vi "expodrive.vi"(10 "Input 2":dbl, 11 "Input":dbl) -> (2 "Output 2":dbl, 3 "Output":dbl)   [LabVIEW 2010, in "LASA Beta.lvrbt"]
uses:
  LASA Beta.lvrbt
  <vilib>/NXT/Dual Mode Library/prims/inRangeAndCoerce/inRangeAndCoerce_int.vi
  <vilib>/NXT/Dual Mode Library/prims/inRangeAndCoerce/inRangeAndCoerce_float.vi
panel:
  in  "Last Sign 2":i32
  in  "Last Sign":i32
  in  "Time 2":i32
  in  "Time 1":i32
  in  "Last Time 2":u32
  in  "Last Time":u32
  # "Time since last update"
  # "Time (ms)"
  # "Last Direction Moved"
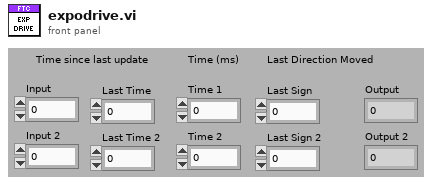
[diagram p1: front panel]
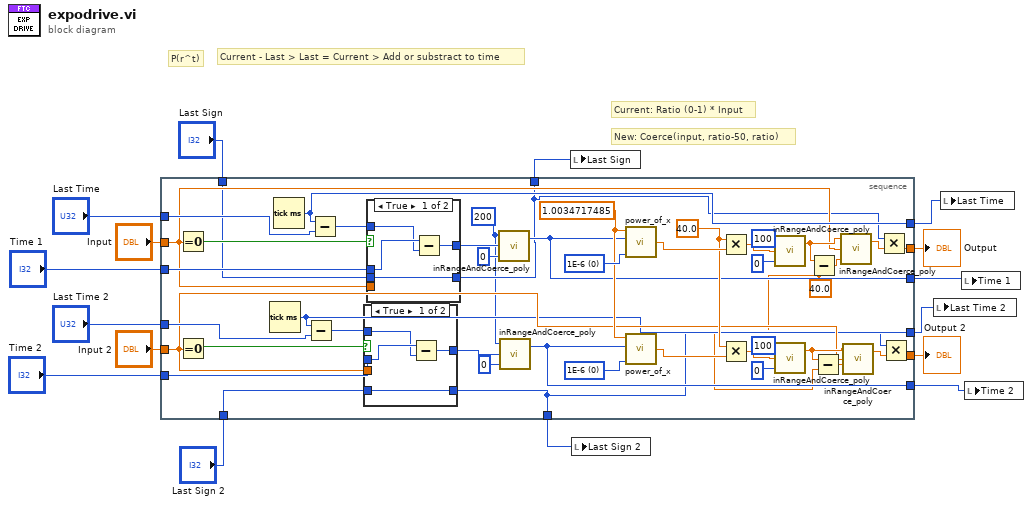
[diagram p0: block diagram]
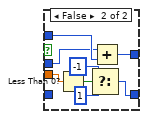
[diagram p2: hidden frame]
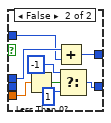
[diagram p3: hidden frame]
diagram:
  # "New: Coerce(input, ratio-50, ratio)"
  # "Current: Ratio (0-1) * Input"
  # "Current - Last > Last = Current > Add or substract to time"
  # "P(r^t)"
  n1 = stacked-sequence {
    tunnel: "Input" -> [w24]
    tunnel: "Input 2" -> [w25]
    tunnel: "Last Time" -> [w47]
    tunnel: [w45] -> w2
    tunnel: "Time 1" -> [w44]
    tunnel: "Last Time 2" -> [w34]
    tunnel: "Time 2" -> [w40]
    tunnel: [w37] -> w4
    tunnel: [w36] -> w3
    tunnel: [w26] -> w10
    tunnel: [w27] -> w9
    tunnel: "Last Sign" -> [w23]
    tunnel: "Last Sign 2" -> [w22]
    tunnel: [w20] -> w6
    tunnel: [w19] -> w5
    tunnel: [w21] -> w1
    frame #0 {
      w17 = 40.0 ("y")
      w18 = 200 ("upper limit")
      w51 = u16 0 items=["1E-6", "1E-5", "1E-4", "1E-3", "1E-2", "1E-1", ""] ("Precision")
      w49 = 40.0
      w56 = u16 0 items=["1E-6", "1E-5", "1E-4", "1E-3", "1E-2", "1E-1", ""] ("Precision")
      w48 = 1.0034717485
      n2 = Equal To 0?(x=w24) -> (x = 0?=w60:bool)
      n3 = Equal To 0?(x=w25) -> (x = 0?=w41:bool)
      n4 = Tick Count (ms)() -> (millisecond timer value=w21:u32)
      n5 = Tick Count (ms)() -> (millisecond timer value=w45:u32)
      n6 = Subtract(x=w21, y=w34) -> (x-y=w35:u32)
      n7 = Subtract(x=w45, y=w47) -> (x-y=w46:u32)
      n8 = case shown="True" w41 {
        tunnel: w35 -> [w63 w72]
        tunnel: w40 -> [w64 w70]
        tunnel: [w62 w71] -> w38
        tunnel: w25 -> [_ w69]
        tunnel: w22 -> [w61 _]
        tunnel: [w61 w65] -> w19
        frame True {
          n9 = Subtract(x=w64, y=w63) -> (x-y=w62:u32)
        }
        frame False {
          n10 = Less Than 0?(x=w69) -> (x < 0?=w68:bool)
          n11 = Select(t=-1, s=w68, f=1) -> (s? t:f=w65:i32)
          n12 = Add(x=w70, y=w72) -> (x+y=w71:u32)
        }
      }
      n13 = case shown="True" w60 {
        tunnel: w46 -> [w75 w83]
        tunnel: w44 -> [w76 w84]
        tunnel: [w74 w82] -> w43
        tunnel: w24 -> [_ w80]
        tunnel: w23 -> [w73 _]
        tunnel: [w73 w79] -> w20
        frame True {
          n14 = Subtract(x=w76, y=w75) -> (x-y=w74:u32)
        }
        frame False {
          n15 = Less Than 0?(x=w80) -> (x < 0?=w81:bool)
          n16 = Add(x=w84, y=w83) -> (x+y=w82:u32)
          n17 = Select(t=-1, s=w81, f=1) -> (s? t:f=w79:i32)
        }
      }
      n18 = call-poly <vilib>:"inRangeAndCoerce_poly.vi"("lower limit"=0, "x"=w43, "upper limit"=w18) -> ("coerced(x)"=w36:i32)  [unwired: 1 out]
      n19 = call-poly <vilib>:"inRangeAndCoerce_poly.vi"("lower limit"=0, "x"=w38, "upper limit"=w18) -> ("coerced(x)"=w37:i32)  [unwired: 1 out]
      n20 = call <vilib>:"power_of_x.vi"("Precision"=w56, "y"=w36, "x"=w48) -> ("x^y"=w55:sgl)  [unwired: 1 in]
      n21 = call <vilib>:"power_of_x.vi"("Precision"=w51, "y"=w37, "x"=w48) -> ("x^y"=w50:sgl)  [unwired: 1 in]
      n22 = Multiply(x=w49, y=w55) -> (x*y=w57:dbl)
      n23 = Multiply(x=w49, y=w50) -> (x*y=w52:dbl)
      n24 = call-poly <vilib>:"inRangeAndCoerce_poly.vi"("lower limit"=0, "x"=w57, "upper limit"=100) -> ("coerced(x)"=w32:dbl)  [unwired: 1 out]
      n25 = call-poly <vilib>:"inRangeAndCoerce_poly.vi"("lower limit"=0, "x"=w52, "upper limit"=100) -> ("coerced(x)"=w29:dbl)  [unwired: 1 out]
      n26 = Subtract(x=w32, y=w17) -> (x-y=w33:dbl)
      n27 = Subtract(x=w29, y=w17) -> (x-y=w30:dbl)
      n28 = call-poly <vilib>:"inRangeAndCoerce_poly.vi"("lower limit"=w33, "x"=w24, "upper limit"=w32) -> ("coerced(x)"=w31:dbl)  [unwired: 1 out]
      n29 = call-poly <vilib>:"inRangeAndCoerce_poly.vi"("lower limit"=w30, "x"=w25, "upper limit"=w29) -> ("coerced(x)"=w28:dbl)  [unwired: 1 out]
      n30 = Multiply(x=w20, y=w31) -> (x*y=w26:dbl)
      n31 = Multiply(x=w19, y=w28) -> (x*y=w27:dbl)
    }
  }
  "Output" <- w10
  "Output 2" <- w9
  n32 = local write "Last Sign"(w6) -> ()
  n33 = local write "Last Sign 2"(w5) -> ()
  n34 = local write "Last Time 2"(w1) -> ()
  n35 = local write "Last Time"(w2) -> ()
  n36 = local write "Time 1"(w3) -> ()
  n37 = local write "Time 2"(w4) -> ()
